vi "Week_4_4.1_Ex-1_Generator-ouput.vi"() -> ()   [LabVIEW 2015]
panel:
  out "3-Phase Genrator O/P":dynamicdata(graph)
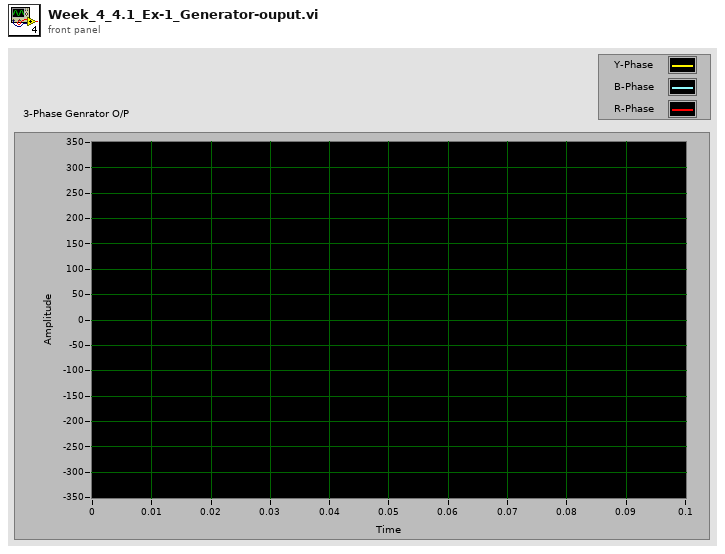
[diagram p1: front panel]
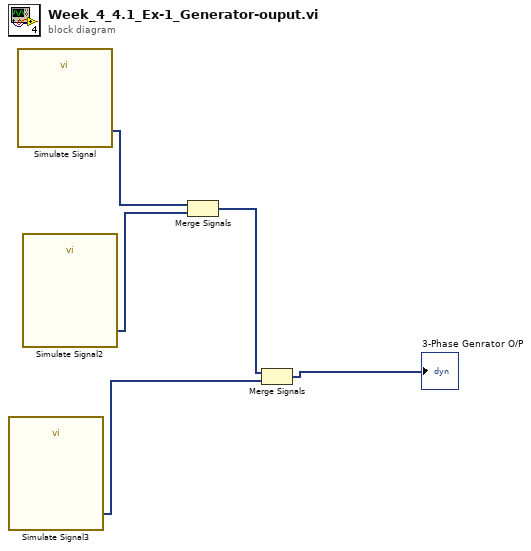
[diagram p0: block diagram]
diagram:
  n1 = call "Simulate Signal3"() -> ("R-Phase"=w3:dynamicdata)  [unwired: 14 in, 1 out]
  n2 = call "Simulate Signal"() -> ("Y-Phase"=w5:dynamicdata)  [unwired: 14 in, 1 out]
  n3 = call "Simulate Signal2"() -> ("B-Phase"=w4:dynamicdata)  [unwired: 14 in, 1 out]
  n4 = Merge Signals(w5, w4) -> (w2:dynamicdata)
  n5 = Merge Signals(w2, w3) -> (→"3-Phase Genrator O/P":dynamicdata)
